vi "GetSurfacePixels.vi"(8 "No Error":errorcluster, 11 "Surface [SDL_Surface *]":i64) -> (0 "error out":errorcluster, 2 "Surface Info":T3 {"flag" items=["SDL_SURFACE_PREALLOCATED"=1, "SDL_SURFACE_LOCK_NEEDED"=2, "SDL_SURFACE_LOCKED"=4, "SDL_SURFACE_SIMD_ALIGNED"=8]}, 3 "Pixels":u8[](array[numeric]) format="%.0x")   [LabVIEW 2024, in "SDL3.lvlib" / "Surface.lvlib"]
doc: "<B>Summary</B>\nRead surface pixels."
uses:
  Surface.lvlib
  SurfaceFlags--ring.ctl
  Pixels/PixelFormat--enum.ctl
  Pixels/Pixels.lvlib
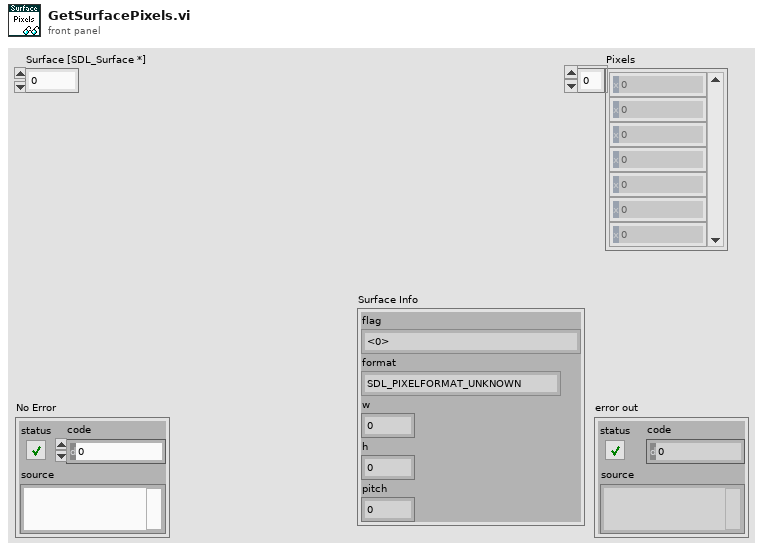
[diagram p1: front panel]
types:
  T1 = typedef "SDL3.lvlib/Surface.lvlib/SurfaceFlags--ring.ctl" = u32
  T2 = typedef "SDL3.lvlib/Pixels.lvlib/PixelFormat--enum.ctl" = enum32{"SDL_PIXELFORMAT_UNKNOWN", "SDL_PIXELFORMAT_INDEX1LSB", "SDL_PIXELFORMAT_INDEX1MSB", "SDL_PIXELFORMAT_INDEX2LSB", "SDL_PIXELFORMAT_INDEX2MSB", "SDL_PIXELFORMAT_INDEX4LSB", "SDL_PIXELFORMAT_INDEX4MSB", "SDL_PIXELFORMAT_INDEX8", "SDL_PIXELFORMAT_RGB332", "SDL_PIXELFORMAT_XRGB4444", "SDL_PIXELFORMAT_XBGR4444", "SDL_PIXELFORMAT_XRGB1555", "SDL_PIXELFORMAT_XBGR1555", "SDL_PIXELFORMAT_ARGB4444", "SDL_PIXELFORMAT_RGBA4444", "SDL_PIXELFORMAT_ABGR4444", "SDL_PIXELFORMAT_BGRA4444", "SDL_PIXELFORMAT_ARGB1555", "SDL_PIXELFORMAT_RGBA5551", "SDL_PIXELFORMAT_ABGR1555", "SDL_PIXELFORMAT_BGRA5551", "SDL_PIXELFORMAT_RGB565", "SDL_PIXELFORMAT_BGR565", "SDL_PIXELFORMAT_RGB24", "SDL_PIXELFORMAT_BGR24", "SDL_PIXELFORMAT_XRGB8888", "SDL_PIXELFORMAT_RGBX8888", "SDL_PIXELFORMAT_XBGR8888", "SDL_PIXELFORMAT_BGRX8888", "SDL_PIXELFORMAT_ARGB8888", "SDL_PIXELFORMAT_RGBA8888", "SDL_PIXELFORMAT_ABGR8888", "SDL_PIXELFORMAT_BGRA8888", "SDL_PIXELFORMAT_XRGB2101010", "SDL_PIXELFORMAT_XBGR2101010", "SDL_PIXELFORMAT_ARGB2101010", "SDL_PIXELFORMAT_ABGR2101010", "SDL_PIXELFORMAT_RGB48", "SDL_PIXELFORMAT_BGR48", "SDL_PIXELFORMAT_RGBA64", "SDL_PIXELFORMAT_ARGB64", "SDL_PIXELFORMAT_BGRA64", "SDL_PIXELFORMAT_ABGR64", "SDL_PIXELFORMAT_RGB48_FLOAT", "SDL_PIXELFORMAT_BGR48_FLOAT", "SDL_PIXELFORMAT_RGBA64_FLOAT", "SDL_PIXELFORMAT_ARGB64_FLOAT", "SDL_PIXELFORMAT_BGRA64_FLOAT", "SDL_PIXELFORMAT_ABGR64_FLOAT", "SDL_PIXELFORMAT_RGB96_FLOAT", "SDL_PIXELFORMAT_BGR96_FLOAT", "SDL_PIXELFORMAT_RGBA128_FLOAT", "SDL_PIXELFORMAT_ARGB128_FLOAT", "SDL_PIXELFORMAT_BGRA128_FLOAT", "SDL_PIXELFORMAT_ABGR128_FLOAT", "SDL_PIXELFORMAT_YV12", "SDL_PIXELFORMAT_IYUV", "SDL_PIXELFORMAT_YUY2", "SDL_PIXELFORMAT_UYVY", "SDL_PIXELFORMAT_YVYU", "SDL_PIXELFORMAT_NV12", "SDL_PIXELFORMAT_NV21", "SDL_PIXELFORMAT_P010", "SDL_PIXELFORMAT_EXTERNAL_OES"}
  T3 = cluster{"flag":T1, "format":T2, "w":i32, "h":i32, "pitch":i32}
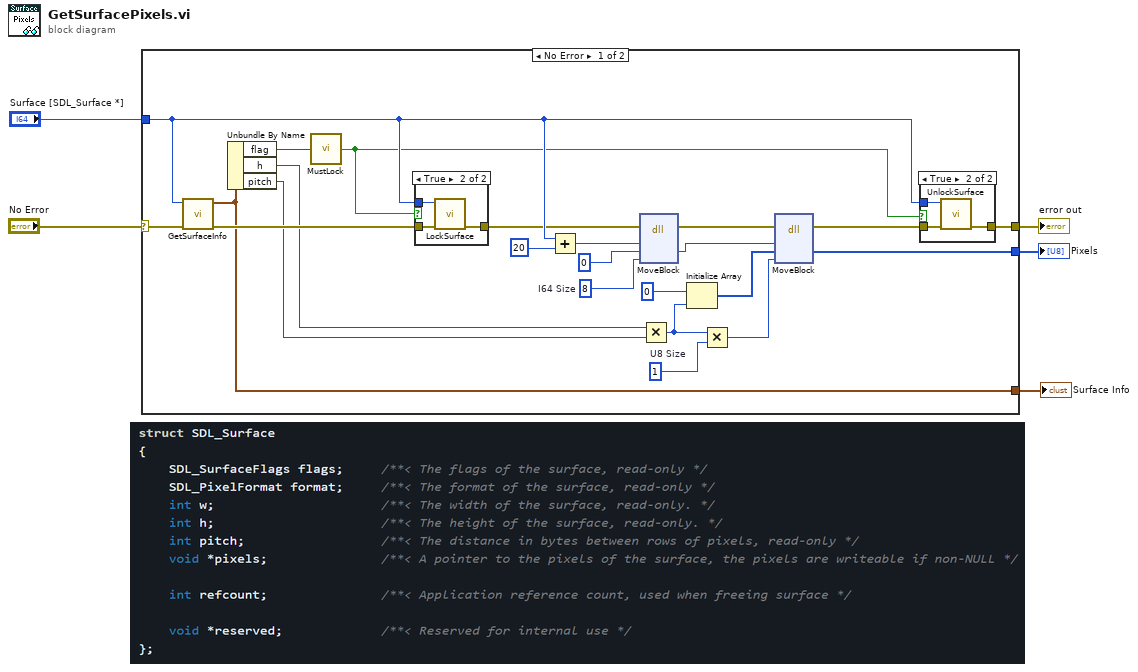
[diagram p0: block diagram]
diagram:
  n1 = case shown="No Error" "No Error" {
    selector: "No Error" -> [w21 w37]
    tunnel: [w18 w37] -> w4
    tunnel: "Surface [SDL_Surface *]" -> [w17 _]
    tunnel: [w23 _] -> w3
    tunnel: [w12 _] -> w1
    frame No Error {
      w8 = 8  # I64 Size
      w24 = 1  # U8 Size
      n2 = call "GetSurfaceInfo.vi"("No Error"=w21, "Surface [SDL_Surface *]"=w17) -> ("error out"=w20:errorcluster, "Surface Info"=w12:T3)  [unwired: 8 in]
      n3 = Unbundle By Name(w12) -> ("flag"=w15:T1, "h"=w14:i32, "pitch"=w13:i32)
      n4 = call "MustLock.vi"("SurfaceFlags"=w15) -> ("Must Lock?"=w16:bool)
      n5 = case shown="True" w16 {
        tunnel: w20 -> [w33 w36]
        tunnel: [w33 w35] -> w11
        tunnel: w17 -> [_ w34]
        frame False {
        }
        frame True {
          n6 = call "LockSurface.vi"("No Error"=w36, "surface [SDL_Surface *]"=w34) -> ("error out"=w35:errorcluster)  [unwired: 9 in]
        }
      }
      n7 = Add(x=w17, y=i64 20) -> (x+y=w9:i64)
      n8 = dll-call lib="LabVIEW" fn="MoveBlock"(error in=w11, "Address"=w9, "Destination"=i64 0, "Size"=w8) -> (error out=w10:errorcluster, "Destination"=w6:i64)  [unwired: 5 in, 1 out]
      n9 = Multiply(x=w14, y=w13) -> (x*y=w22:i32)
      n10 = Initialize Array(u8 0, w22) -> (w27:u8[])
      n11 = Multiply(x=w22, y=w24) -> (x*y=w25:i32)
      n12 = dll-call lib="LabVIEW" fn="MoveBlock"(error in=w10, "Address"=w6, "Destination"=w27, "Size"=w25) -> (error out=w19:errorcluster, "Destination"=w23:u8[])  [unwired: 5 in, 1 out]
      n13 = case shown="True" w16 {
        tunnel: w19 -> [w29 w32]
        tunnel: [w29 w31] -> w18
        tunnel: w17 -> [_ w30]
        frame False {
        }
        frame True {
          n14 = call "UnlockSurface.vi"("No Error"=w32, "surface [SDL_Surface *]"=w30) -> ("error out"=w31:errorcluster)  [unwired: 9 in]
        }
      }
    }
    frame Error {
    }
  }
  "error out" <- w4
  "Pixels" <- w3
  "Surface Info" <- w1
